vi "SV Spectrum Info Probe.vi"(1 "spectrum info":T3 {"x-axis units" items=["Time (s)"=0, "Frequency-CB (Hz)"=1, "Frequency-CPB (Hz)"=1248, "Frequency-Arbitrary (Hz)"=2357, "Quefrency (s)"=2, "Revolutions (rev)"=3, "Order"=4, "Speed (RPM)"=11, "Speed (rad/s)"=21, "Index"=65535]; "weighting filter" items=["Linear", "A-weighting", "B-weighting", "C-weighting", "ITU-R 468-4", "Dolby", "CCITT", "C-message", "Wb", "Wc", "Wd", "We", "Wf", "Wh", "Wj", "Wk", "Wm", "AES17 20 kHz lowpass", "AES17 40 kHz lowpass", "AES17 20 kHz highpass", "AES17 40 kHz highpass"]; "dB reference [EU]" format="%.2f"; "engineering units" items=["custom..."=0, "V"=1, "A"=21, "C"=30, "pC"=31, "s"=32, "-"=29, "Pa"=2, "N"=20, "g"=3, "m/s^2"=4, "m/s"=5, "m"=6, "mm/s"=12, "mm"=13, "micron/s"=14, "micron"=15, "in/s^2"=7, "in/s"=8, "in"=9, "mil/s"=10, "mil"=11, "rad/s^2"=16, "rad/s"=17, "rad"=18, "deg/s^2"=26, "deg/s"=27, "deg"=28, "RPM"=22, "cycle/s^2"=23, "Hz"=24, "cycle"=25, "strain"=19]; "spectral info"."window" items=["None "=0, "Hanning"=1, "Hamming"=2, "Blackman-Harris"=3, "Exact Blackman"=4, "Blackman"=5, "Flat Top"=6, "4 Term B-Harris "=7, "7 Term B-Harris"=8, "Low Sidelobe"=9, "Force - Exponential"=10, "Gaussian"=62]}) -> (0 "Boolean":bool)   [LabVIEW 2017]
uses:
  <vilib>/addons/_NISVFA/_Shared subVIs/Controls/svc_Spectrum Info.ctl
  <vilib>/addons/_NISVFA/_Shared subVIs/Controls/svc_X-Axis Units.ctl
  <vilib>/addons/_NISVFA/_Shared subVIs/Controls/svc_Spectrum Type.ctl
  <vilib>/addons/_NISVFA/_Shared subVIs/Controls/svc_Engineering Units Text Ring.ctl
  <vilib>/addons/_NISVFA/_Shared subVIs/Controls/svc_Weighting Filter Text Ring.ctl
  <vilib>/addons/_NISVFA/_Shared subVIs/Controls/svc_Complimentary Spectrum Units.ctl
  <vilib>/addons/_NISVFA/_Shared subVIs/Controls/NI Spectrum Component.ctl
panel:
  out "y2-axis label":string
  out "y2-axis unit label":string
  out "phase unwrapped":bool
  out "y-axis label":string
  out "x-axis unit label":string
  out "orders to track":dbl[](array[numeric])
  out "window parameter":dbl format="%.2f"
  out "spectrum skewed":bool
  out "spectral density":bool
  out "complimentary spectrum (y2) units":T1(ring)
  out "x-axis label":string
  out "peak units":enum16{"rms", "peak", "peak-peak"}(ring)
  out "weighting filter":u16(ring) items=["Linear", "A-weighting", "B-weighting", "C-weighting", "ITU-R 468-4", "Dolby", "CCITT", "C-message"]
  out "custom label":string
  out "dB reference [EU]":dbl format="%#_3p"
  out "engineering units":u16(ring) items=["custom..."=0, "V"=1, "A"=21, "Pa"=2, "N"=20, "g"=3, "m/s^2"=4, "m/s"=5, "m"=6, "mm/s"=12, "mm"=13, "microns/s"=14, "microns"=15, "in/s^2"=7, "in/s"=8, "in"=9, "mils/s"=10, "mils"=11, "rad/s^2"=16, "rad/s"=17, "rad"=18, "strain"=19]
  out "FFT size":i32
  out "window size":i32
  out "window":u16(ring) items=["None "=0, "Hanning"=1, "Hamming"=2, "Blackman-Harris"=3, "Exact Blackman"=4, "Blackman"=5, "Flat Top"=6, "4 Term B-Harris "=7, "7 Term B-Harris"=8, "Low Sidelobe"=9, "Force - Exponential"=10, "Gaussian"=62]
  out "linear/dB":enum16{"linear", "dB"}(ring)
  out "spectrum type":T2(ring)
  out "y-axis unit label":string
  out "description":string
  out "channel name":string
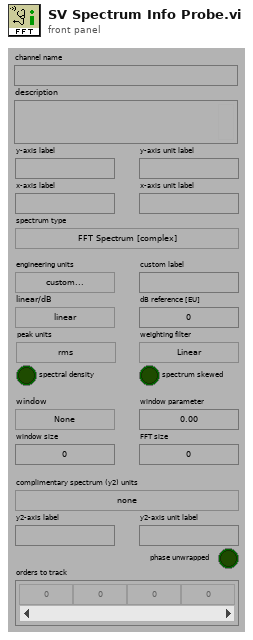
[diagram p1: front panel]
types:
  T1 = enum16{"none", "radians", "degrees", "cycles", "imaginary"}
  T2 = enum16{"FFT Spectrum [complex]", "Amplitude [Magnitude]", "Power [Magnitude^2]", "Cross Spectrum [complex]", "Frequency Response [Complex]"}
  T3 = typedef "svc_Spectrum Info.ctl" = cluster{"channel name":string, "description":string, "x-axis units":T4, "spectral info":cluster{"spectrum type":T5, "linear/dB":enum16{"linear", "dB"}, "window":u16, "window size":i32, "FFT size":i32}, "engineering units":T6, "custom label":string, "dB reference [EU]":dbl, "peak units":enum16{"rms", "peak", "peak-peak"}, "weighting filter":T7, "spectral density?":bool, "unit label":string, "spectrum skewed?":bool, "complimentary spectrum units":T8}
  T4 = typedef "svc_X-Axis Units.ctl" = u16
  T5 = typedef "svc_Spectrum Type.ctl" = enum16{"FFT Spectrum [complex]", "Amplitude [Magnitude]", "Power [Magnitude^2]", "Cross Spectrum [complex]", "Frequency Response [Complex]"}
  T6 = typedef "svc_Engineering Units Text Ring.ctl" = u16
  T7 = typedef "svc_Weighting Filter Text Ring.ctl" = u16
  T8 = typedef "svc_Complimentary Spectrum Units.ctl" = enum16{"none", "radians", "degrees", "cycles", "imaginary"}
  T9 = typedef "NI Spectrum Component.ctl" = u16
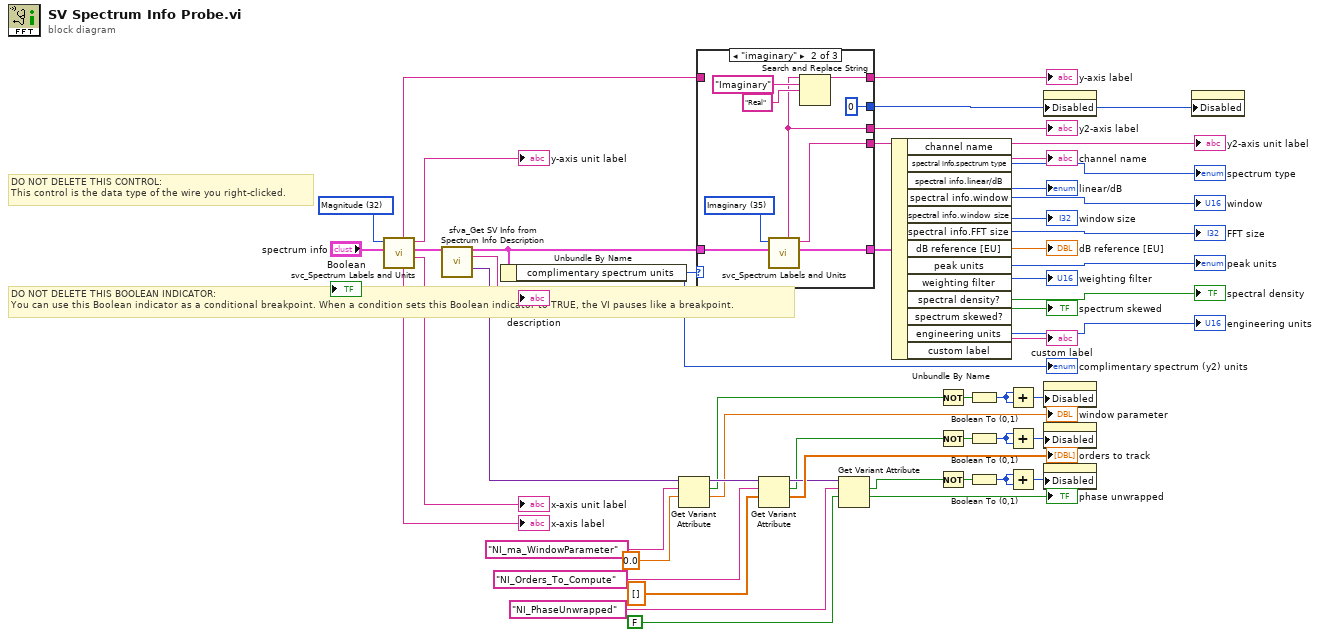
[diagram p0: block diagram]
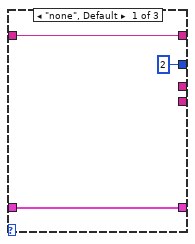
[diagram p2: hidden frame]
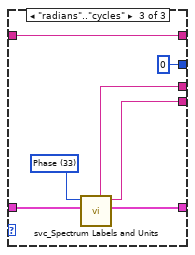
[diagram p3: hidden frame]
diagram:
  w47 = T9 32 items=["Magnitude"=32, "Phase"=33, "Real"=34, "Imaginary"=35, "Coherence"=36, "Unknown"=99] ("spectrum component")
  # "DO NOT DELETE THIS BOOLEAN INDICATOR: \nYou can use this Boolean indicator as a conditional breakpoint. When a condition sets this Boolean indicator to TRUE, the VI pauses like a breakpoint."
  # "DO NOT DELETE THIS CONTROL: \nThis control is the data type of the wire you right-clicked."
  n1 = call <vilib>:"svc_Spectrum Labels and Units.vi"("spectrum info in"="spectrum info", "spectrum component"=w47) -> ("x-axis unit label"=→"x-axis unit label":string, "spectrum info out"=w51:T3, "unit label"=→"y-axis unit label":string, "x-axis label"=→"x-axis label":string, "y-axis label"=w45:string)  [unwired: 4 in, 1 out]
  n2 = call <vilib>:"sfva_Get SV Info from Spectrum Info Description.vi"("spectrum info"=w51) -> ("spectrum info"=w40:T3, "description"=→"description":string, "SV Info"=w20:variant)  [unwired: 10 in, 2 out]
  n3 = Unbundle By Name(w40) -> ("complimentary spectrum units"=w39:T8)
  "complimentary spectrum (y2) units" <- w39
  n4 = Get Variant Attribute(Variant=w20, name="NI_ma_WindowParameter", default value (empty Variant)=0.0 ("window parameter")) -> (duplicate Variant=w19:variant, found=w17:bool, value=→"window parameter":dbl)  [unwired: 1 in, 1 out]
  n5 = case shown="\"imaginary\"" w39 {
    tunnel: w45 -> [w55 _ w71]
    tunnel: [w55 w62 w71] -> w44
    tunnel: w40 -> [w54 w63 w70]
    tunnel: [w54 w59 w68] -> w43
    tunnel: [_ w58 w66] -> w5
    tunnel: [_ w57 w67] -> w4
    tunnel: [u8 2 ("Disabled") u8 0 ("Disabled") u8 0 ("Disabled")] -> w3
    frame "none", Default {
    }
    frame "imaginary" {
      w64 = T9 35 items=["Magnitude"=32, "Phase"=33, "Real"=34, "Imaginary"=35, "Coherence"=36, "Unknown"=99] ("spectrum component")
      n6 = call <vilib>:"svc_Spectrum Labels and Units.vi"("spectrum info in"=w63, "spectrum component"=w64) -> ("spectrum info out"=w59:T3, "unit label"=w58:string, "y-axis label"=w57:string)  [unwired: 4 in, 3 out]
      n7 = Search and Replace String(input string=w57, search string="Imaginary", replace string="Real" ("replace string (\"\")")) -> (result string=w62:string)  [unwired: 5 in, 3 out]
    }
    frame "radians".."cycles" {
      w69 = T9 33 items=["Magnitude"=32, "Phase"=33, "Real"=34, "Imaginary"=35, "Coherence"=36, "Unknown"=99] ("spectrum component")
      n8 = call <vilib>:"svc_Spectrum Labels and Units.vi"("spectrum info in"=w70, "spectrum component"=w69) -> ("spectrum info out"=w68:T3, "unit label"=w66:string, "y-axis label"=w67:string)  [unwired: 4 in, 3 out]
    }
  }
  "y-axis label" <- w44
  "y2-axis unit label" <- w5
  "y2-axis label" <- w4
  n9 = Get Variant Attribute(Variant=w19, name="NI_Orders_To_Compute", default value (empty Variant)=dbl[] [] ("orders to track")) -> (duplicate Variant=w21:variant, found=w7:bool, value=→"orders to track":dbl[])  [unwired: 1 in, 1 out]
  n10 = Get Variant Attribute(Variant=w21, name="NI_PhaseUnwrapped", default value (empty Variant)=FALSE ("dB on? (F)")) -> (found=w9:bool, value=→"phase unwrapped":bool)  [unwired: 1 in, 2 out]
  n11 = Unbundle By Name(w43) -> ("channel name"=→"channel name":string, "spectral info.spectrum type"=→"spectrum type":T5, "spectral info.linear/dB"=→"linear/dB":enum16{"linear", "dB"}, "spectral info.window"=→"window":u16, "spectral info.window size"=→"window size":i32, "spectral info.FFT size"=→"FFT size":i32, "dB reference [EU]"=→"dB reference [EU]":dbl, "peak units"=→"peak units":enum16{"rms", "peak", "peak-peak"}, "weighting filter"=→"weighting filter":T7, "spectral density?"=→"spectral density":bool, "spectrum skewed?"=→"spectrum skewed":bool, "engineering units"=→"engineering units":T6, "custom label"=→"custom label":string)
  n12 = Not(x=w17) -> (.not. x?=w12:bool)
  n13 = Not(x=w7) -> (.not. x?=w13:bool)
  n14 = Not(x=w9) -> (.not. x?=w10:bool)
  n15 = Boolean To (0,1)(Boolean=w12) -> (0, 1=w16:i16)
  n16 = Boolean To (0,1)(Boolean=w13) -> (0, 1=w14:i16)
  n17 = Boolean To (0,1)(Boolean=w10) -> (0, 1=w11:i16)
  n18 = Add(x=w16, y=w16) -> (x+y=w15:i16)
  n19 = Add(x=w14, y=w14) -> (x+y=w6:i16)
  n20 = Add(x=w11, y=w11) -> (x+y=w8:i16)
  n21 = property on="y2-axis label" class="Str"("Disabled"=w3) -> ()  [unwired: 2 in, 2 out]
  n22 = property on="window parameter" class="DigNum (strict)"("Disabled"=w15) -> ()  [unwired: 2 in, 2 out]
  n23 = property on="orders to track" class="Arr (strict)"("Disabled"=w6) -> ()  [unwired: 2 in, 2 out]
  n24 = property on="phase unwrapped" class="Bool (strict)"("Disabled"=w8) -> ()  [unwired: 2 in, 2 out]
  n25 = property on="y2-axis unit label" class="Str"("Disabled"=w3) -> ()  [unwired: 2 in, 2 out]
